vi "Filter 1D Array Example 01.vi"() -> ()   [LabVIEW 2019]
uses:
  user.lib/_OpenG.lib/array/array.llb/Filter 1D Array (String)__ogtk.vi
panel:
  out "Filtered Array":string[](array[string])
  in  "Items to Filter":string[](array[string])=["Apple", "Monkey"]
  in  "Array":string[](array[string])=["Pear", "Apple", "Monkey", "Fish", "Monkey", "Apple", "Fish"]
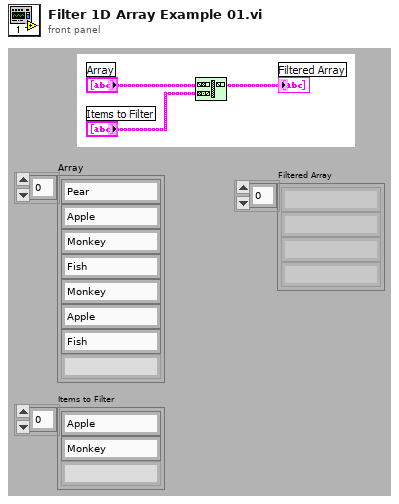
[diagram p1: front panel]
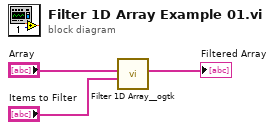
[diagram p0: block diagram]
diagram:
  n1 = call-poly "Filter 1D Array__ogtk.vi"("items to filter"="Items to Filter", "array"="Array") -> ("filtered array"=→"Filtered Array":string[])  [unwired: 4 in, 1 out]
